vi "access_as_address.vi"(9 "column number":i32, 10 "row number":i32, 11 "Array":dbl[][](array[numeric])) -> (3 "subarray":dbl[](array[numeric]))   [LabVIEW 2014]
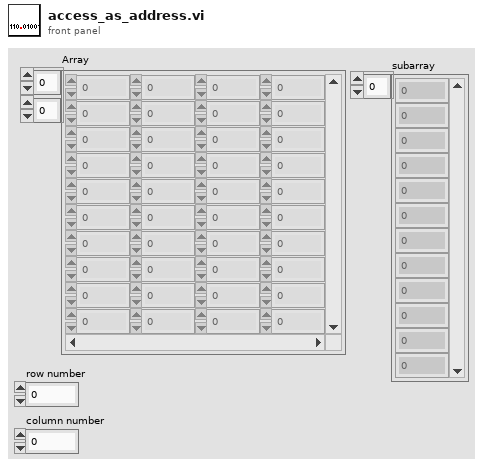
[diagram p1: front panel]
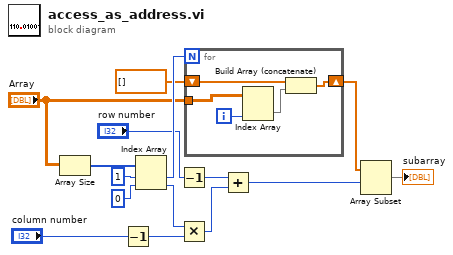
[diagram p0: block diagram]
diagram:
  n1 = Array Size(array="Array") -> (size(s)=w15:i32[])
  n2 = Decrement(x="column number") -> (x-1=w5:i32)
  n3 = Index Array(array=w15, index #1=1 ("index"), index #2=0 ("index")) -> (element #1=w14:i32, element #2=w9:i32)
  n4 = Decrement(x="row number") -> (x-1=w4:i32)
  n5 = Multiply(x=w9, y=w5) -> (x*y=w8:i32)
  n6 = for {
    N: w14 -> [_]
    tunnel: "Array" -> [w20]
    shift-right: [w18] -> w7
    shift-left: dbl[] [] -> [w17]
    i -> [w16]
    n7 = Index Array(array=w20, index (col)=w16) -> (element=w19:dbl[])  [unwired: 1 in]
    n8 = Build Array (concatenate)(w17, w19) -> (w18:dbl[])
  }
  n9 = Add(x=w4, y=w8) -> (x+y=w3:i32)
  n10 = Array Subset(array=w7, index=w3) -> (→"subarray":dbl[])  [unwired: 1 in]
